vi "Test settings dialog.vi"(8 "error in (no error)":errorcluster, 11 "LIVE DATA 3":refnum<vi>) -> (0 "error out":errorcluster, 2 "Confirmed":bool, 3 "Test identifier out":string)   [LabVIEW 2016]
uses:
  Controls/Test settings.ctl
  Actuator/Controls/Actuator fgv modes.ctl
  <vilib>/Utility/inputDevices.llb/keyboardAcquire.vi
  <vilib>/Utility/inputDevices.llb/closeKeyboard.vi
panel:
  in  "Time interval (s)":dbl=0.5 caption="s" min=0.5
  in  "Snap intervals":bool caption="Active"
  in  "Test notes":string
  in  "Send trigger":bool
  out "Position.Y":dbl
  in  "Wait on trigger":bool caption="Trigger"
  in  "Wait time (s)":dbl=2.0 caption="s" min=0.0
  in  "Time wait":bool=TRUE caption="Active"
  in  "Test settings":T1={"Speed (mm/s)"=0.0001, "Position limit"=FALSE, "Position limit (mm)"=0.0001, "Load limit"=FALSE, "Load limit (N)"=0.0001, "No. of repeats"=0, "Test identifier"="", "Time wait"=FALSE, "Wait time (s)"=0.0, "Trigger wait"=FALSE, "Send trigger"=FALSE, "Test notes"="", "Snap intervals"=FALSE, "Time interval (s)"=0.5} {"Time interval (s)" min=0.5; "No. of repeats" min=1 max=20 step=1; "Load limit (N)" min=0.0001 max=20.0 step=0.0001; "Position limit (mm)" min=0.0001 max=20.0 step=0.0001; "Speed (mm/s)" min=0.0001 max=20.0 step=0.0001}
  in  "No. of repeats":u16 min=1 max=20 step=1
  in  "Load limit":bool caption="Active"
  in  "Position limit":bool=TRUE caption="Active"
  in  "Load limit (N)":dbl=0.0001 caption="N" min=0.0001 max=20.0 step=0.0001
  in  "Position limit (mm)":dbl=10.0 caption="mm" min=0.0001 max=100.0 step=0.0001
  in  "Speed (mm/s)":dbl=0.0001 caption="mm/s" min=0.0001 max=20.0 step=0.0001
  in  "Confirm":bool
  in  "Cancel":bool
  in  "Test identifier":string
  # "TEST SETTINGS"
  # "File ID"
  # "Test speed"
  # "Stop conditions"
  # "Return after"
  # "Output"
  # "Camera snap interval"
  # "Notes"
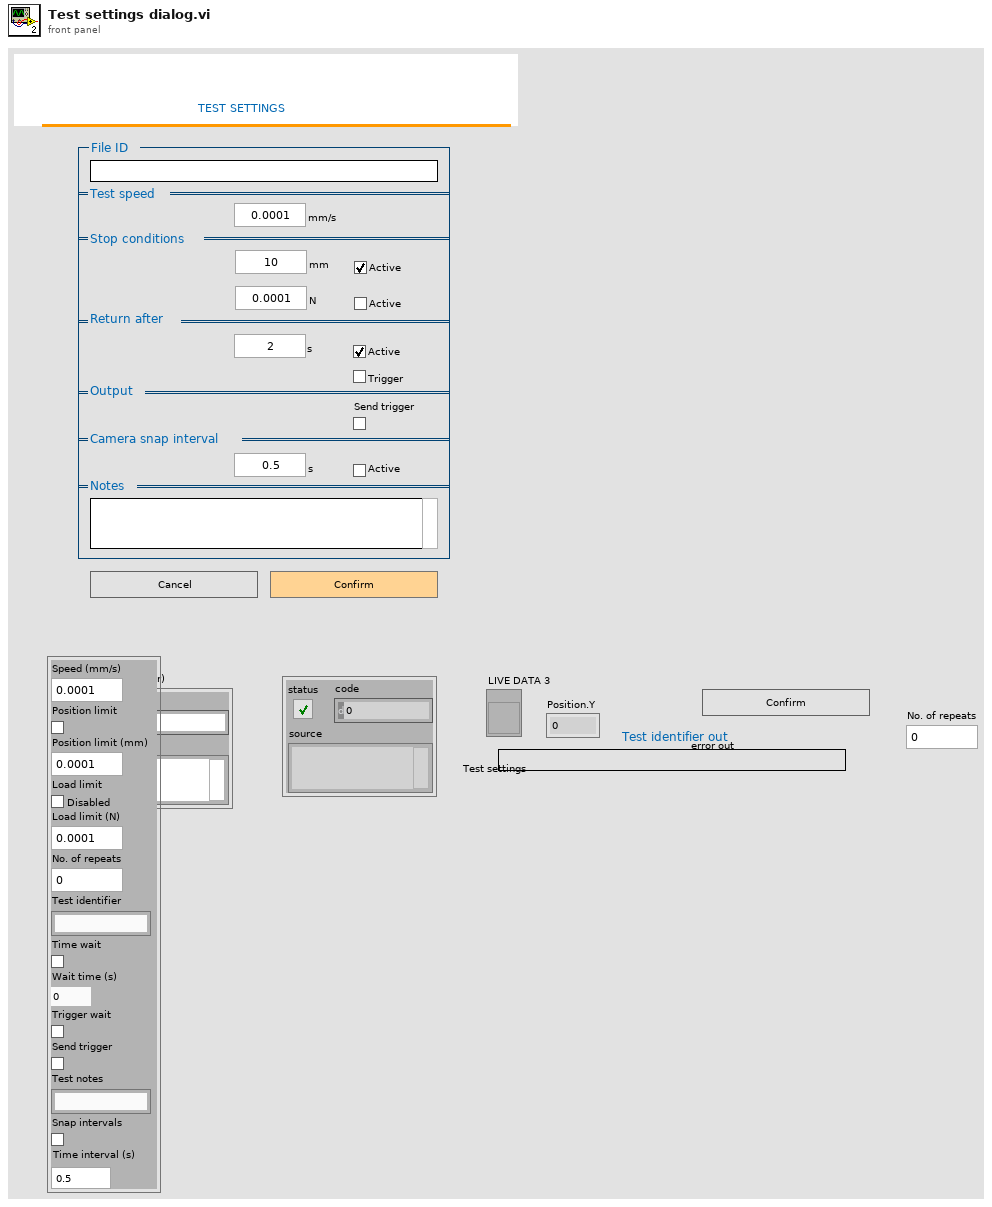
[diagram p1: front panel]
types:
  T1 = typedef "Test settings.ctl" = cluster{"Speed (mm/s)":dbl, "Position limit":bool, "Position limit (mm)":dbl, "Load limit":bool, "Load limit (N)":dbl, "No. of repeats":u16, "Test identifier":string, "Time wait":bool, "Wait time (s)":dbl, "Trigger wait":bool, "Send trigger":bool, "Test notes":string, "Snap intervals":bool, "Time interval (s)":dbl}
  T2 = typedef "LVCursorListTypeDef.ctl" = cluster{"Name":string, "Color":u32, "Style":u8, "Point Style":u8, "Name Visible":bool, "Allow Drag":bool, "Cursor Mode":u32, "Plot":i32, "Index":i32, "Position":cluster{"X":dbl, "Y":dbl}, "X Scale":u32, "Y Scale":u32, "Watch Plots":i32[], "Watch All Plots":bool, "Plot Area":i32, "Label Offset":cluster{"X":dbl, "Y":dbl}}[]
  T3 = typedef "References.ctl" = cluster{"Tab Control":refnum<vi>, "Logo 1":refnum<vi>, "Logo 2":refnum<vi>, "Connect Actuator":refnum<vi>, "LIVE DATA":refnum<vi>, "Speed":refnum<vi>, "Home position":refnum<vi>, "Limit position":refnum<vi>, "Trigger":refnum<vi>, "Current position":refnum<vi>, "Connect Camera":refnum<vi>, "TEST DATA":refnum<vi>, "LIVE DATA Force":refnum<vi>, "Connect DAQ":refnum<vi>, "Initialised":refnum<vi>, "Test":refnum<vi>}
  T4 = cluster{"Name":string, "Color":u32, "Style":u8, "Point Style":u8, "Name Visible":bool, "Allow Drag":bool, "Cursor Mode":u32, "Plot":i32, "Index":i32, "Position":cluster{"X":dbl, "Y":dbl}, "X Scale":u32, "Y Scale":u32, "Watch Plots":i32[], "Watch All Plots":bool, "Plot Area":i32, "Label Offset":cluster{"X":dbl, "Y":dbl}}
  T5 = typedef "Actuator fgv modes.ctl" = enum16{"Initalise", "COM", "Limit", "Speed", "Home", "Get"}
  T6 = enum16{"0", "1", "2", "3", "4", "5", "6", "7", "8", "9", "A", "B", "C", "D", "E", "F", "G", "H", "I", "J", "K", "L", "M", "N", "O", "P", "Q", "R", "S", "T", "U", "V", "W", "X", "Y", "Z", "F1", "F2", "F3", "F4", "F5", "F6", "F7", "F8", "F9", "F10", "F11", "F12", "F13", "F14", "F15", "ADD", "BACK", "BACKSLASH", "CAPITAL", "COMMA", "DECIMAL", "DELETE", "DIVIDE", "DOWN", "END", "EQUALS", "ESCAPE", "GRAVE (`)", "HOME", "INSERT", "LBRACKET", "LCONTROL", "LEFT", "L ALT", "LSHIFT", "LWIN", "MINUS", "MULTIPLY", "NEXT", "NUMLOCK", "NUMPAD_0", "NUMPAD_1", "NUMPAD_2", "NUMPAD_3", "NUMPAD_4", "NUMPAD_5", "NUMPAD_6", "NUMPAD_7", "NUMPAD_8", "NUMPAD_9", "PAUSE", "PERIOD", "PRIOR (PG UP)", "RBRACKET", "RCONTROL", "RETURN", "RIGHT", "R ALT", "RSHIFT", "RWIN", "SCROLL", "SEMICOLON", "SLASH", "SPACE", "SUBTRACT", "TAB", "UP", "ENTER (num pad)", "' (quote)"}
  T7 = enum16{"0", "1", "2", "3", "4", "5", "6", "7", "8", "9", "A", "B", "C", "D", "E", "F", "G", "H", "I", "J", "K", "L", "M", "N", "O", "P", "Q", "R", "S", "T", "U", "V", "W", "X", "Y", "Z", "F1", "F2", "F3", "F4", "F5", "F6", "F7", "F8", "F9", "F10", "F11", "F12", "F13", "F14", "F15", "ADD", "BACK", "BACKSLASH", "CAPITAL", "COMMA", "DECIMAL", "DELETE", "DIVIDE", "DOWN", "END", "EQUALS", "ESCAPE", "GRAVE (`)", "HOME", "INSERT", "LBRACKET", "LCONTROL", "LEFT", "L ALT", "LSHIFT", "LWIN", "MINUS", "MULTIPLY", "NEXT", "NUMLOCK", "NUMPAD_0", "NUMPAD_1", "NUMPAD_2", "NUMPAD_3", "NUMPAD_4", "NUMPAD_5", "NUMPAD_6", "NUMPAD_7", "NUMPAD_8", "NUMPAD_9", "PAUSE", "PERIOD", "PRIOR (PG UP)", "RBRACKET", "RCONTROL", "RETURN", "RIGHT", "R ALT", "RSHIFT", "RWIN", "SCROLL", "SEMICOLON", "SLASH", "SPACE", "SUBTRACT", "TAB", "UP", "ENTER (num pad)", "' (quote)"}[]
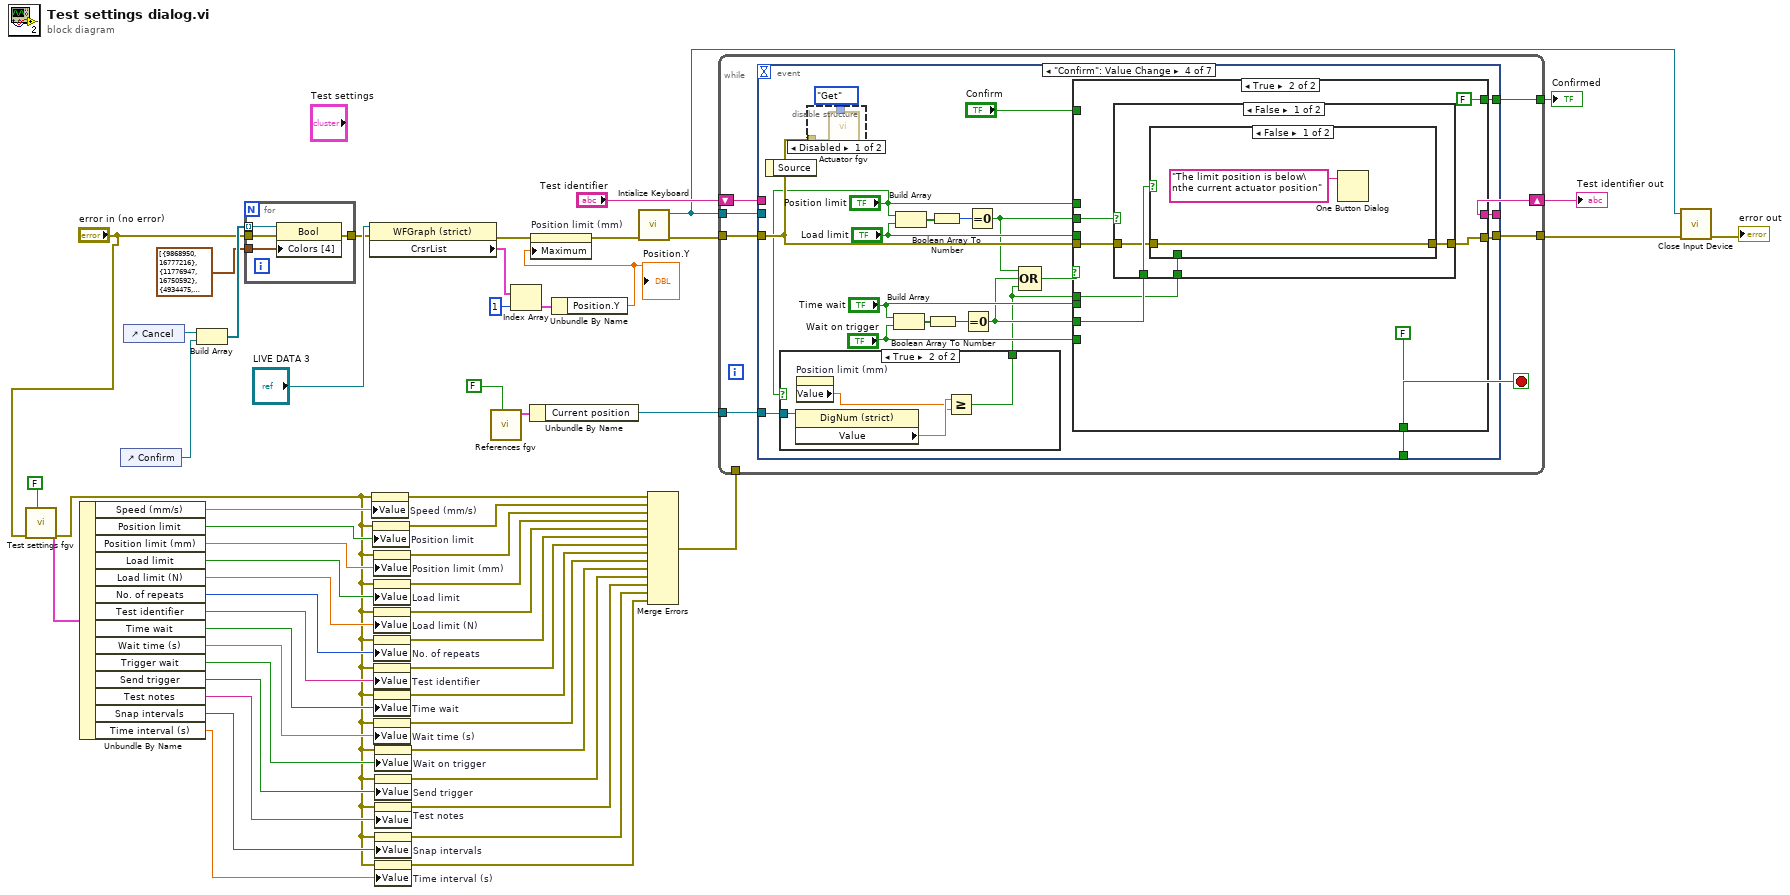
[diagram p0: block diagram]
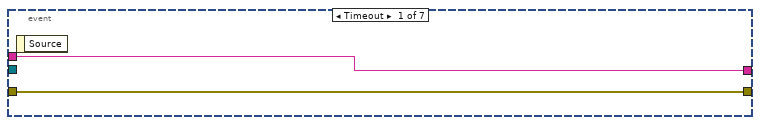
[diagram p2: hidden frame]
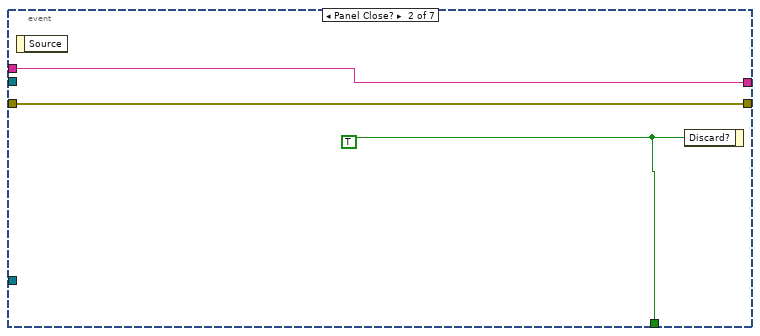
[diagram p3: hidden frame]
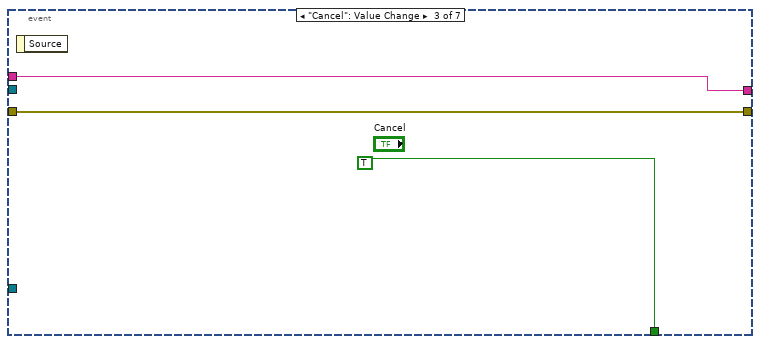
[diagram p4: hidden frame]
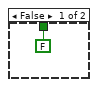
[diagram p5: hidden frame]
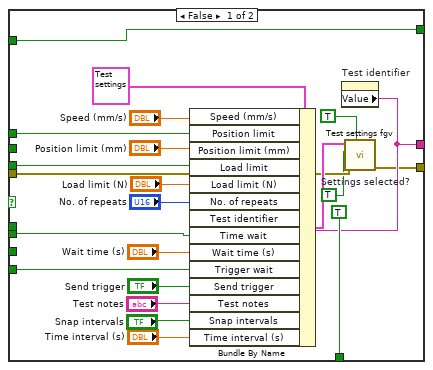
[diagram p6: hidden frame]
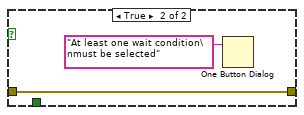
[diagram p7: hidden frame]
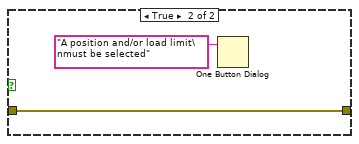
[diagram p8: hidden frame]
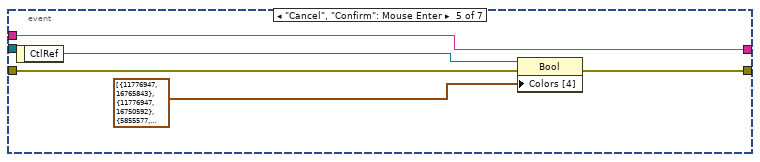
[diagram p10: hidden frame]
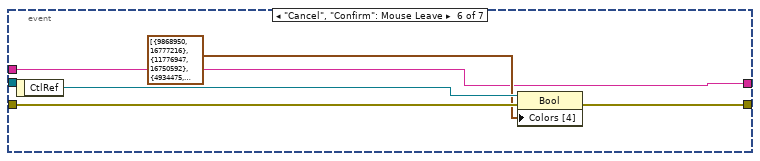
[diagram p11: hidden frame]
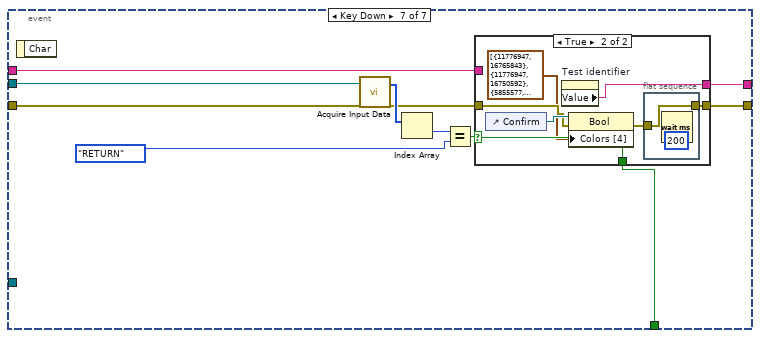
[diagram p12: hidden frame]
diagram:
  n1 = call "Test settings fgv.vi"("Set?"=FALSE, "error in (no error)"="error in (no error)") -> ("error out"=w7:errorcluster, "Test settings out"=w36:T1)  [unwired: 7 in, 1 out]
  n2 = Unbundle By Name(w36) -> ("Speed (mm/s)"=w34:dbl, "Position limit"=w33:bool, "Position limit (mm)"=w32:dbl, "Load limit"=w31:bool, "Load limit (N)"=w30:dbl, "No. of repeats"=w29:u16, "Test identifier"=w28:string, "Time wait"=w27:bool, "Wait time (s)"=w26:dbl, "Trigger wait"=w25:bool, "Send trigger"=w11:bool, "Test notes"=w10:string, "Snap intervals"=w8:bool, "Time interval (s)"=w6:dbl)
  n3 = control-ref of="Confirm"() -> (w54:refnum<vi>)
  n4 = control-ref of="Cancel"() -> (w55:refnum<vi>)
  n5 = Build Array(w55, w54) -> (w53:refnum<vi>[])
  n6 = for {
    tunnel: "error in (no error)" -> [w59]
    tunnel: [w58] -> w42
    tunnel: w53 -> [w57] mode=indexing
    tunnel: cluster{u32, u32}[] [{9868950, 16777216}, {11776947, 16750592}, {4934475, 16777216}, {5855577, 8342528}] ("Colors [4]") -> [w56]
    n7 = property class="Bool"(reference=w57, error in=w59, "Colors [4]"=w56) -> (error out=w58:errorcluster)  [unwired: 1 out]
  }
  n8 = property class="WFGraph (strict)"(reference="LIVE DATA 3", error in=w42) -> (error out=w38:errorcluster, "CrsrList"=w44:T2)  [unwired: 1 out]
  n9 = property on="Speed (mm/s)" class="DigNum (strict)"(error in=w7, "Value"=w34) -> (error out=w24:errorcluster)  [unwired: 1 in, 1 out]
  n10 = property on="Position limit" class="Bool (strict)"(error in=w7, "Value"=w33) -> (error out=w23:errorcluster)  [unwired: 1 in, 1 out]
  n11 = property on="Position limit (mm)" class="DigNum (strict)"(error in=w7, "Value"=w32) -> (error out=w22:errorcluster)  [unwired: 1 in, 1 out]
  n12 = property on="Load limit" class="Bool (strict)"(error in=w7, "Value"=w31) -> (error out=w21:errorcluster)  [unwired: 1 in, 1 out]
  n13 = property on="Load limit (N)" class="DigNum (strict)"(error in=w7, "Value"=w30) -> (error out=w20:errorcluster)  [unwired: 1 in, 1 out]
  n14 = property on="No. of repeats" class="DigNum (strict)"(error in=w7, "Value"=w29) -> (error out=w19:errorcluster)  [unwired: 1 in, 1 out]
  n15 = property on="Test identifier" class="Str"(error in=w7, "Value"=w28) -> (error out=w18:errorcluster)  [unwired: 1 in, 1 out]
  n16 = property on="Time wait" class="Bool (strict)"(error in=w7, "Value"=w27) -> (error out=w17:errorcluster)  [unwired: 1 in, 1 out]
  n17 = property on="Wait time (s)" class="DigNum (strict)"(error in=w7, "Value"=w26) -> (error out=w16:errorcluster)  [unwired: 1 in, 1 out]
  n18 = property on="Wait on trigger" class="Bool (strict)"(error in=w7, "Value"=w25) -> (error out=w15:errorcluster)  [unwired: 1 in, 1 out]
  n19 = property on="Send trigger" class="Bool (strict)"(error in=w7, "Value"=w11) -> (error out=w12:errorcluster)  [unwired: 1 in, 1 out]
  n20 = property on="Test notes" class="Str"(error in=w7, "Value"=w10) -> (error out=w9:errorcluster)  [unwired: 1 in, 1 out]
  n21 = property on="Snap intervals" class="Bool (strict)"(error in=w7, "Value"=w8) -> (error out=w5:errorcluster)  [unwired: 1 in, 1 out]
  n22 = property on="Time interval (s)" class="DigNum (strict)"(error in=w7, "Value"=w6) -> (error out=w4:errorcluster)  [unwired: 1 in, 1 out]
  n23 = call "References fgv.vi"("Set?"=FALSE) -> ("Cluster"=w2:T3)  [unwired: 9 in, 1 out]
  n24 = Index Array(array=w44, index=1) -> (element=w40:T4)
  n25 = Unbundle By Name(w2) -> ("Current position"=w1:refnum<vi>)
  n26 = Unbundle By Name(w40) -> ("Position.Y"=w39:dbl)
  "Position.Y" <- w39
  n27 = property on="Position limit (mm)" class="DigNum (strict)"(error in=w38, "Maximum"=w39) -> (error out=w45:errorcluster)  [unwired: 1 in, 1 out]
  n28 = call <vilib>:"Intialize Keyboard.vi"("error in (no error)"=w45) -> ("error out"=w49:errorcluster, "device ID"=w46:refnum<k1>)  [unwired: 9 in]
  n29 = Merge Errors(w24, w23, w22, w21, w20, w19, w18, w17, w16, w15, w12, w9, w5, w4) -> (w14:errorcluster)
  n30 = while {
    tunnel: w49 -> [w66]
    tunnel: [w65] -> w47
    shift-right: [w63] -> w50
    shift-left: "Test identifier" -> [w64]
    tunnel: w46 -> [w62]
    tunnel: [w61] -> w37
    tunnel: w14 -> [_]
    tunnel: w1 -> [w60]
    stop <- w67 stop-if-true
    n31 = event shown="[3] \"Confirm\": Value Change" {
      selector: _ -> [_ _ _ _ _ _ _]
      dyn-events: _ -> [_ _ _ _ _ _ _]
      timeout: _ -> [_ _ _ _ _ _ _]
      tunnel: [_ w72 TRUE ("Discard?") w95 _ _ w156] -> w67
      tunnel: w66 -> [w69 w71 w74 w92 w145 w151 w162]
      tunnel: [w69 w71 w74 w93 w144 w150 w152] -> w65
      tunnel: [w68 w70 w73 w94 w142 w147 w154] -> w63
      tunnel: w64 -> [w68 w70 w73 _ w142 w147 w155]
      tunnel: w62 -> [_ _ _ _ _ _ w161]
      tunnel: [_ _ _ w90 _ _ _] -> w61
      tunnel: w60 -> [_ _ _ w78 _ _ _]
      event Timeout {
        n32 = event-data() -> ()  [unwired: 1 in, 1 out]
      }
      event Panel Close? {
        w72 = TRUE ("Discard?")
        n33 = event-data() -> ()  [unwired: 1 in, 1 out]
        n34 = event-data("Discard?"=w72) -> ()  [unwired: 1 in, 1 out]
      }
      event "Cancel": Value Change {
        n35 = event-data() -> ()  [unwired: 1 in, 1 out]
      }
      event "Confirm": Value Change {
        n36 = event-data() -> ()  [unwired: 1 in, 1 out]
        n37 = case shown="True" "Position limit" {
          tunnel: w78 -> [_ w100]
          tunnel: [FALSE w97] -> w76
          frame False {
          }
          frame True {
            n38 = property class="DigNum (strict)"(reference=w100) -> ("Value"=w99:dbl)  [unwired: 1 in, 2 out]
            n39 = property on="Position limit (mm)" class="DigNum (strict)"() -> ("Value"=w98:dbl)  [unwired: 2 in, 2 out]
            n40 = Greater Or Equal?(x=w99, y=w98) -> (x >= y?=w97:bool)
          }
        }
        n41 = disable-structure shown="Disabled" {
          disable-tunnel: w92 -> [w141 _]
          disable-tunnel: Actuator_fgv_modes."Get" ("Enum") -> [w140 _]
          frame Disabled {
            n42 = call "Actuator fgv.vi"("Enum"=w140, "error in (no error)"=w141) -> ()  [unwired: 8 in, 2 out]
          }
          frame Enabled {
          }
        }
        n43 = Build Array("Time wait", "Wait on trigger") -> (w86:bool[])
        n44 = Build Array("Position limit", "Load limit") -> (w85:bool[])
        n45 = Boolean Array To Number(Boolean array=w86) -> (number=w83:u32)
        n46 = Boolean Array To Number(Boolean array=w85) -> (number=w84:u32)
        n47 = Equal To 0?(x=w83) -> (x = 0?=w80:bool)
        n48 = Equal To 0?(x=w84) -> (x = 0?=w81:bool)
        n49 = Compound Arithmetic op=OR(w81, w80, w76) -> (w82:bool)
        n50 = case shown="True" w82 {
          tunnel: [TRUE ("Discard?") FALSE ("Discard?")] -> w95
          tunnel: [w117 _] -> w94
          tunnel: [w116 w124] -> w93
          tunnel: w92 -> [w113 w125]
          tunnel: [w105 FALSE ("Confirm")] -> w90
          tunnel: "Time wait" -> [w109 _]
          tunnel: "Wait on trigger" -> [w108 _]
          tunnel: "Position limit" -> [w107 _]
          tunnel: "Load limit" -> [w106 _]
          tunnel: w81 -> [_ w127]
          tunnel: w80 -> [_ w126]
          tunnel: "Confirm" -> [w105 _]
          tunnel: w76 -> [_ w123]
          frame False {
            w111 = TRUE  # Settings selected?
            n51 = property on="Test identifier" class="Str"() -> ("Value"=w117:string)  [unwired: 2 in, 2 out]
            n52 = Bundle By Name(cluster=T1 {"Speed (mm/s)"=0.0001, "Position limit"=FALSE, "Position limit (mm)"=0.0001, "Load limit"=FALSE, "Load limit (N)"=0.0001, "No. of repeats"=0, "Test identifier"="", "Time wait"=FALSE, "Wait time (s)"=0.0, "Trigger wait"=FALSE, "Send trigger"=FALSE, "Test notes"="", "Snap intervals"=FALSE, "Time interval (s)"=0.5} ("Test settings"), "Speed (mm/s)"="Speed (mm/s)", "Position limit"=w107, "Position limit (mm)"="Position limit (mm)", "Load limit"=w106, "Load limit (N)"="Load limit (N)", "No. of repeats"="No. of repeats", "Test identifier"=w117, "Time wait"=w109, "Wait time (s)"="Wait time (s)", "Trigger wait"=w108, "Send trigger"="Send trigger", "Test notes"="Test notes", "Snap intervals"="Snap intervals", "Time interval (s)"="Time interval (s)") -> (w115:T1)
            n53 = call "Test settings fgv.vi"("Set?"=TRUE, "error in (no error)"=w113, "Settings selected?"=w111, "Test settings"=w115) -> ("error out"=w116:errorcluster)  [unwired: 5 in, 2 out]
          }
          frame True {
            n54 = case shown="False" w127 {
              tunnel: w126 -> [w133 _]
              tunnel: w125 -> [w132 w138]
              tunnel: [w131 w138] -> w124
              tunnel: w123 -> [w130 _]
              frame False {
                n55 = case shown="False" w133 {
                  tunnel: w132 -> [w135 w136]
                  tunnel: [w135 w136] -> w131
                  tunnel: w130 -> [_ _]
                  frame False {
                    n56 = One Button Dialog(message="The limit position is below\nthe current actuator position") -> ()  [unwired: 1 in, 1 out]
                  }
                  frame True {
                    n57 = One Button Dialog(message="At least one wait condition\nmust be selected") -> ()  [unwired: 1 in, 1 out]
                  }
                }
              }
              frame True {
                n58 = One Button Dialog(message="A position and/or load limit\nmust be selected") -> ()  [unwired: 1 in, 1 out]
              }
            }
          }
        }
      }
      event "Cancel", "Confirm": Mouse Enter {
        n59 = event-data() -> ("CtlRef"=w143:refnum<vi>)  [unwired: 1 in]
        n60 = property class="Bool"(reference=w143, error in=w145, "Colors [4]"=cluster{u32, u32}[] [{11776947, 16765843}, {11776947, 16750592}, {5855577, 8350025}, {5855577, 8342528}]) -> (error out=w144:errorcluster)  [unwired: 1 out]
      }
      event "Cancel", "Confirm": Mouse Leave {
        n61 = event-data() -> ("CtlRef"=w149:refnum<vi>)  [unwired: 1 in]
        n62 = property class="Bool"(reference=w149, error in=w151, "Colors [4]"=cluster{u32, u32}[] [{9868950, 16777216}, {11776947, 16750592}, {4934475, 16777216}, {5855577, 8342528}]) -> (error out=w150:errorcluster)  [unwired: 1 out]
      }
      event Key Down {
        n63 = event-data() -> ()  [unwired: 1 in, 1 out]
        n64 = call-poly <vilib>:"Acquire Input Data.vi"("device ID"=w161, "error in (no error)"=w162) -> ("keys pressed"=w160:T7, "error out"=w153:errorcluster)  [unwired: 15 in, 1 out]
        n65 = Index Array(array=w160) -> (element=w159:T6)  [unwired: 1 in]
        n66 = Equal?(x=w159, y=T6."RETURN" ("keyType 3")) -> (x = y?=w157:bool)
        n67 = case shown="True" w157 {
          selector: w157 -> [w163 w172]
          tunnel: [w163 w172] -> w156
          tunnel: w155 -> [w165 _]
          tunnel: [w165 w171] -> w154
          tunnel: w153 -> [w164 w169]
          tunnel: [w164 w166] -> w152
          frame False {
          }
          frame True {
            n68 = control-ref of="Confirm"() -> (w170:refnum<vi>)
            n69 = property on="Test identifier" class="Str"() -> ("Value"=w171:string)  [unwired: 2 in, 2 out]
            n70 = property class="Bool"(reference=w170, error in=w169, "Colors [4]"=cluster{u32, u32}[] [{11776947, 16765843}, {11776947, 16750592}, {5855577, 8350025}, {5855577, 8342528}]) -> (error out=w167:errorcluster)  [unwired: 1 out]
            n71 = flat-sequence {
              tunnel: w167 -> [w173]
              tunnel: [w173] -> w166
              frame #0 {
                n72 = Wait (ms)(milliseconds to wait=u32 200) -> ()  [unwired: 1 out]
              }
            }
          }
        }
      }
    }
  }
  "Test identifier out" <- w50
  "Confirmed" <- w37
  n73 = call-poly <vilib>:"Close Input Device.vi"("error in (no error)"=w47, "device ID"=w46) -> ("error out"=→"error out":errorcluster)  [unwired: 8 in]
